vi "getScriptoObjFromClassName_core.vi"(8 "error in (no error)":errorcluster, 11 "className":string) -> (0 "error out":errorcluster, 1 "found?":bool, 3 "matchingObj":refnum<class "Generic.lvclass">)   [LabVIEW 2023, in "TLC_Scripto.lvlib"]
uses:
  TLC_Scripto.lvlib
  Generic/Generic.lvclass
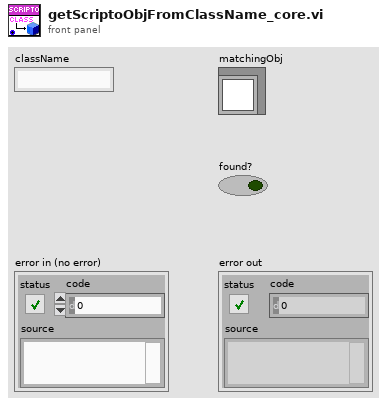
[diagram p1: front panel]
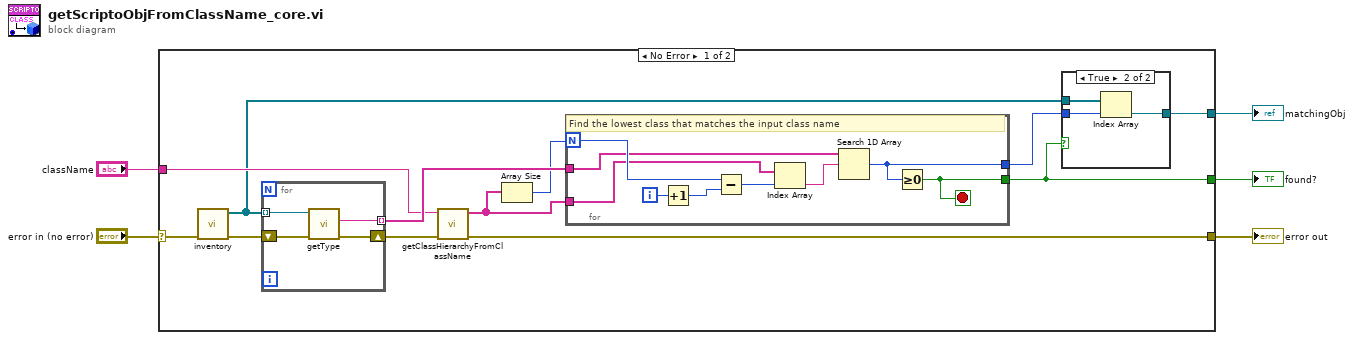
[diagram p0: block diagram]
diagram:
  n1 = case shown="No Error" "error in (no error)" {
    selector: "error in (no error)" -> [w12 w34]
    tunnel: [w17 w34] -> w5
    tunnel: [w6 _] -> w1
    tunnel: [w9 _] -> w4
    tunnel: "className" -> [w14 _]
    frame No Error {
      n2 = call "inventory.vi"("error in"=w12) -> ("error out"=w13:errorcluster, "classList"=w7:refnum<class "Generic.lvclass">[])  [unwired: 7 in, 2 out]
      n3 = for {
        tunnel: w7 -> [w24] mode=indexing
        shift-right: [w22] -> w15
        shift-left: w13 -> [w23]
        tunnel: [w21] -> w16 mode=indexing
        n4 = call-dynamic "getType.vi"("error in (no error)"=w23, "Generic In"=w24) -> ("error out"=w22:errorcluster, "type"=w21:string)  [unwired: 7 in, 1 out]
      }
      n5 = call "getClassHierarchyFromClassName.vi"("error in (no error)"=w15, "className"=w14) -> ("error out"=w17:errorcluster, "hierarchy"=w10:string[])  [unwired: 8 in]
      n6 = Array Size(array=w10) -> (size(s)=w11:i32)
      n7 = for {
        N: w11 -> [w33]
        tunnel: w10 -> [w30]
        tunnel: w16 -> [w29]
        tunnel: [w25] -> w9
        tunnel: [w27] -> w8
        i -> [w32]
        stop <- w25 stop-if-true
        # "Find the lowest class that matches the input class name"
        n8 = Increment(x=w32) -> (x+1=w31:i32)
        n9 = Subtract(x=w33, y=w31) -> (x-y=w28:i32)
        n10 = Index Array(array=w30, index=w28) -> (element=w26:string)
        n11 = Search 1D Array(1D array=w29, element=w26) -> (index of element=w27:i32)  [unwired: 1 in]
        n12 = Greater Or Equal To 0?(x=w27) -> (x >= 0?=w25:bool)
      }
      n13 = case shown="True" w9 {
        tunnel: w8 -> [_ w19]
        tunnel: w7 -> [_ w20]
        tunnel: [_ w18] -> w6
        frame False {
        }
        frame True {
          n14 = Index Array(array=w20, index=w19) -> (element=w18:refnum<class "Generic.lvclass">)
        }
      }
    }
    frame Error {
    }
  }
  "error out" <- w5
  "found?" <- w4
  "matchingObj" <- w1
